vi "[GV]_Lidar Obstacle.vi"() -> ()   [LabVIEW 2016, in "Lidar Variables.lvlib"]
uses:
  Lidar Variables.lvlib
panel:
  out "LIDAR Obstacle":dbl[][](array[numeric])
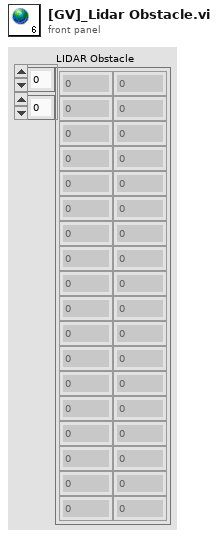
[diagram p1: front panel]
diagram:
